vi "SingleCounter - Readout.vi"(8 "Error In":errorcluster, 10 "seconds to wait":dbl=0.1 format="%.3f", 11 "task in":refnum<k21>) -> (0 "error out":errorcluster, 1 "counts":i32, 2 "time tags":u32[](array[numeric]))   [LabVIEW 2018]
uses:
  <vilib>/Utility/error.llb/DialogType.ctl
  <vilib>/DAQmx/read.llb/DAQmx Read (Counter 1D U32 1Chan NSamp).vi
  <vilib>/DAQmx/miscellaneous.llb/DAQmx Fill In Error Info.vi
  Global_variables.vi
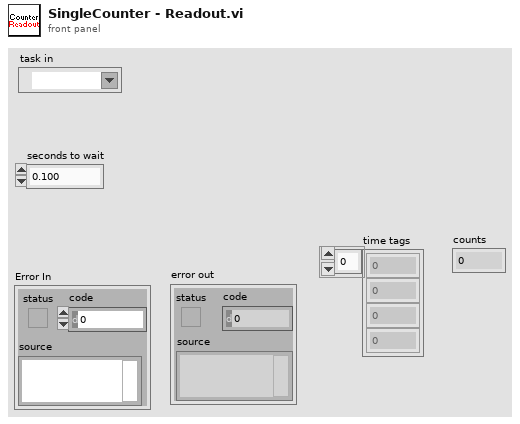
[diagram p1: front panel]
types:
  T1 = typedef "DialogType.ctl" = u16
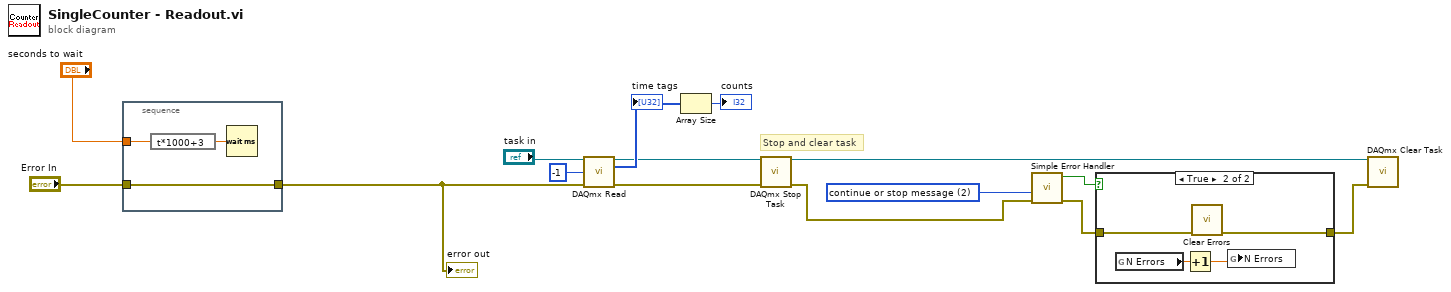
[diagram p0: block diagram]
diagram:
  w4 = T1 2 items=["no dialog", "OK message", "continue or stop message", "OK message + warnings", "continue/stop + warnings"] ("type of dialog (OK msg:1)")
  # "Stop and clear task"
  n1 = stacked-sequence {
    tunnel: "Error In" -> [w18]
    tunnel: [w18] -> w9
    tunnel: "seconds to wait" -> [w16]
    frame #0 {
      n2 = expression code="t*1000+3"(w16) -> (w17:dbl)
      n3 = Wait (ms)(milliseconds to wait=w17) -> ()  [unwired: 1 out]
    }
  }
  "error out" <- w9
  n4 = call-poly <vilib>:"DAQmx Read.vi"("task/channels in"="task in", "number of samples per channel"=-1 ("Samples per Channel \n(-1 for all samples)"), "error in"=w9) -> ("task out"=w7:refnum<k21>, "data"=w11:u32[], "error out"=w6:errorcluster)  [unwired: 10 in]
  "time tags" <- w11
  n5 = Array Size(array=w11) -> (size(s)=→"counts":i32)
  n6 = call <vilib>:"DAQmx Stop Task.vi"("task/channels in"=w7, "error in"=w6) -> ("task out"=w15:refnum<k21>, "error out"=w5:errorcluster)  [unwired: 12 in]
  n7 = call <vilib>:"Simple Error Handler.vi"("type of dialog (OK msg:1)"=w4, "error in (no error)"=w5) -> ("error?"=w3:bool, "error out"=w2:errorcluster)  [unwired: 3 in, 3 out]
  n8 = case shown="True" w3 {
    tunnel: [w19 w22] -> w1
    tunnel: w2 -> [w19 w23]
    frame False {
    }
    frame True {
      n9 = global read "Global_variables.vi" "N Errors"() -> (w21:dbl)
      n10 = Increment(x=w21) -> (x+1=w20:dbl)
      n11 = call <vilib>:"Clear Errors.vi"("error in (no error)"=w23) -> ("error out"=w22:errorcluster)  [unwired: 5 in, 1 out]
      n12 = global write "Global_variables.vi" "N Errors"(w20) -> ()
    }
  }
  n13 = call <vilib>:"DAQmx Clear Task.vi"("task in"=w15, "error in"=w1) -> ()  [unwired: 13 in, 1 out]
